vi "SetRTC.vi"(8 "error in (no error)":errorcluster, 10 "RTC":timestamp, 11 "reference in":refnum<class "Flux_Capacitor.lvclass">) -> (0 "error out":errorcluster, 1 "OK":bool, 3 "reference in":refnum<class "Flux_Capacitor.lvclass">)   [LabVIEW 2022 SP3, in "Flux_Capacitor.lvlib" / "Flux_Capacitor.lvclass"]
uses:
  Flux_Capacitor.lvclass
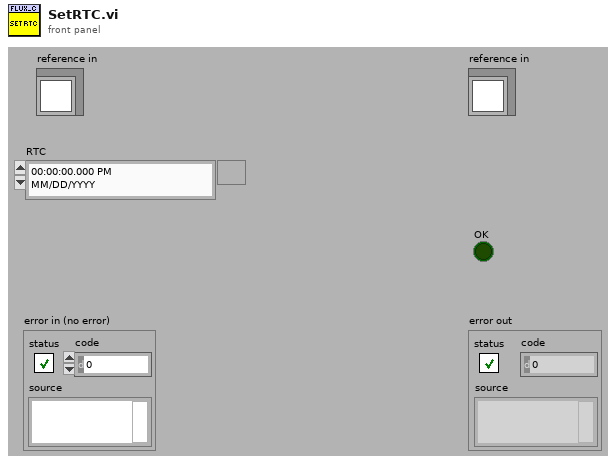
[diagram p1: front panel]
types:
  T1 = typedef "Flux_Capacitor.lvlib/Flux_Capacitor.lvclass/ObjectAttributes.ctl" = cluster{"Config":T2, "T Sensors":T3[], "Temp_DegC":dbl[], "Temp_Raw":u64[], "RTC":timestamp, "Flux":bool, "Time":timestamp, "RTC_Live":timestamp}
  T2 = typedef "Flux_Capacitor.lvlib/Flux_Capacitor.lvclass/Config.ctl" = cluster{"default":string}
  T3 = typedef "Flux_Capacitor.lvlib/Flux_Capacitor.lvclass/TempSensor.ctl" = enum16{"1", "2", "3"}
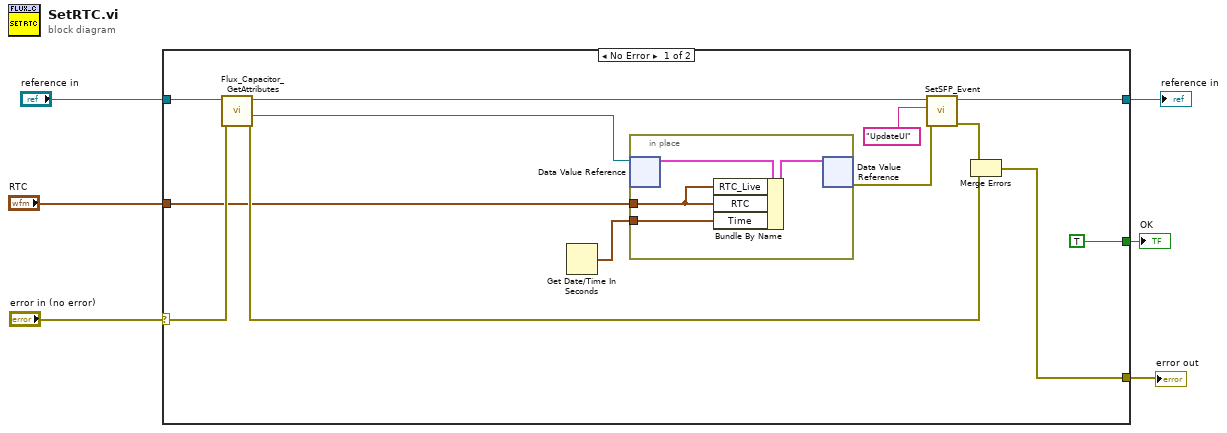
[diagram p0: block diagram]
diagram:
  n1 = case shown="No Error" "error in (no error)" {
    selector: "error in (no error)" -> [w19 w25]
    tunnel: [w11 w25] -> w3
    tunnel: [w10 w24] -> w2
    tunnel: "reference in" -> [w18 w24]
    tunnel: [TRUE _] -> w1
    tunnel: "RTC" -> [w8 _]
    frame No Error {
      n2 = call "Flux_Capacitor_GetAttributes.vi"("error in (no error)"=w19, "reference in"=w18) -> ("error out"=w13:errorcluster, "DataRef"=w14:refnum<data-value>, "reference out"=w12:refnum<class "Flux_Capacitor.lvclass">)  [unwired: 6 in, 1 out]
      n3 = Get Date/Time In Seconds() -> (seconds since 1Jan1904=w7:timestamp)
      n4 = in-place {
        in-place-border: w7 -> [w21]
        in-place-border: w8 -> [w20]
        n5 = in-place-dvr #1(w14) -> (w23:T1)  [unwired: 1 out]
        n6 = Bundle By Name(cluster=w23, "RTC_Live"=w20, "RTC"=w20, "Time"=w21) -> (w22:T1)
        n7 = in-place-dvr #1(w22) -> (w17:errorcluster)  [unwired: 1 out]
      }
      n8 = call-dynamic "SetSFP_Event.vi"("error in (no error)"=w17, "msg"="UpdateUI", "reference in"=w12) -> ("error out"=w16:errorcluster, "reference out"=w10:refnum<class "Flux_Capacitor.lvclass">)  [unwired: 7 in]
      n9 = Merge Errors(w16, w13) -> (w11:errorcluster)
    }
    frame Error {
    }
  }
  "error out" <- w3
  "reference in" <- w2
  "OK" <- w1
